vi "Get_Alias_Table.vi"(1 "API Functions Table":cluster{string, string, path}[](array[cluster]), 2 "Alias Table In":string[][](array[string])) -> (0 "Alias Table Out":string[][](array[string]))   [LabVIEW 2011]
doc: "This VI takes the \"API Functions Table\" parameter and appends those API Function aliases to the supplied \"Alias Table\"."
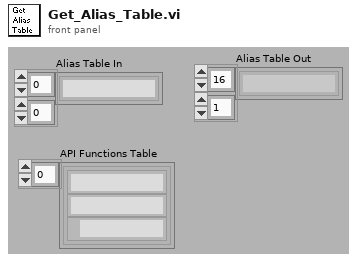
[diagram p1: front panel]
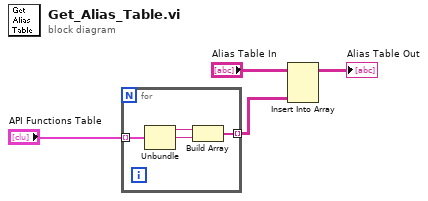
[diagram p0: block diagram]
diagram:
  n1 = for {
    tunnel: "API Functions Table" -> [w8] mode=indexing
    tunnel: [w5] -> w4 mode=indexing
    n2 = Unbundle(w8) -> (w7:string, w6:string)  [unwired: 1 out]
    n3 = Build Array(w7, w6) -> (w5:string[])
  }
  n4 = Insert Into Array(array="Alias Table In", new element=w4) -> (→"Alias Table Out":string[][])  [unwired: 2 in]
